vi "AuMT8852B AFH Scale.vi"(5 "Scale Factor (10)":enum16{"10", "20", "50", "100"}(ring), 7 "Set/Get (Set)":enum16{"Set", "Get"}(ring)=enum."Get", 8 "error in (no error)":errorcluster, 11 "VISA session":refnum<visa-resource-name>) -> (0 "error out":errorcluster, 2 "error code":i32, 3 "VISA session out":refnum<visa-resource-name>, 4 "Scale Factor out":enum16{"10", "20", "50", "100"}(ring))   [LabVIEW 2017]
doc: "Anritsu MT8852B Bluetooth Tester\n\nControls the scale value used for the \"chart recorder\" display when measuring channel utilisation or FER.\n\nINPUTS\nSet/Get - whether the value is being sent to or retrieved from the instrument.\nScale Factor - chart recorder display scale factor (10, 20, 50 and 100) setting.\n\nOUTPUTS\nScale Factor out - current chart recorder display scale setting."
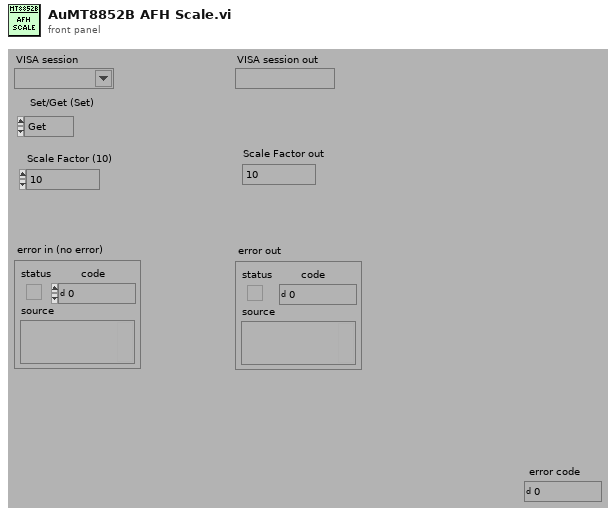
[diagram p1: front panel]
types:
  T1 = enum16{"Simulate", "Range check", "Cache", "Query instrument status"}
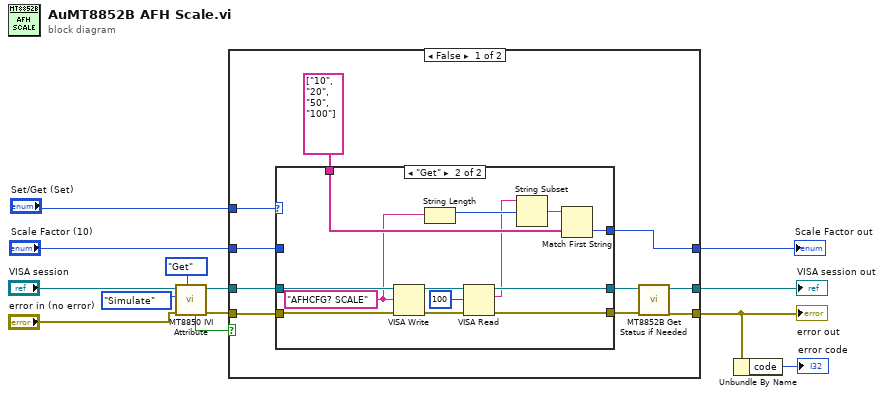
[diagram p0: block diagram]
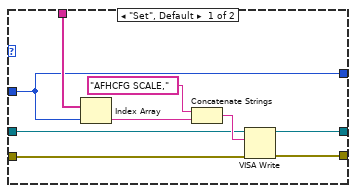
[diagram p2: hidden frame]
diagram:
  n1 = call <instrlib>:"MT8850 IVI Attribute.vi"("Set/Get (Set)"=enum16{"Set", "Get"}."Get", "error in (no error)"="error in (no error)", "Flag (Simulate)"=T1."Simulate", "VISA session"="VISA session") -> ("error out"=w12:errorcluster, "VISA session out"=w13:refnum<visa-resource-name>, "Value out"=w9:bool)  [unwired: 5 in]
  n2 = case shown="False" w9 {
    tunnel: [w18 w48] -> w7
    tunnel: [w19 w47] -> w6
    tunnel: w13 -> [w20 w48]
    tunnel: w12 -> [w21 w47]
    tunnel: [w22 w46] -> w3
    tunnel: "Scale Factor (10)" -> [w15 w46]
    tunnel: "Set/Get (Set)" -> [w14 _]
    frame False {
      n3 = case shown="\"Get\"" w14 {
        tunnel: string[] ["10", "20", "50", "100"] -> [w32 w42]
        tunnel: w15 -> [w28 _]
        tunnel: [w28 w41] -> w22
        tunnel: [w24 w38] -> w16
        tunnel: [w25 w37] -> w17
        tunnel: w21 -> [w27 w40]
        tunnel: w20 -> [w26 w39]
        frame "Set", Default {
          n4 = Index Array(array=w32, index=w28) -> (element=w31:string)
          n5 = Concatenate Strings("AFHCFG SCALE," ("write buffer (\"\")"), w31) -> (w29:string)
          n6 = VISA Write(VISA resource name=w26, write buffer=w29, error in (no error)=w27) -> (VISA resource name out=w25:refnum<visa-resource-name>, error out=w24:errorcluster)  [unwired: 1 out]
        }
        frame "Get" {
          w36 = "AFHCFG? SCALE" ("write buffer (\"\")")
          n7 = VISA Write(VISA resource name=w39, write buffer=w36, error in (no error)=w40) -> (VISA resource name out=w44:refnum<visa-resource-name>, error out=w45:errorcluster)  [unwired: 1 out]
          n8 = String Length(string=w36) -> (length=w34:i32)
          n9 = VISA Read(VISA resource name=w44, byte count=u32 100 ("byte count (0)"), error in (no error)=w45) -> (VISA resource name out=w37:refnum<visa-resource-name>, read buffer=w33:string, error out=w38:errorcluster)  [unwired: 1 out]
          n10 = String Subset(string=w33, offset (0)=w34) -> (substring=w35:string)  [unwired: 1 in]
          n11 = Match First String(2:w42, 3:w35) -> (0:w41:i32)  [unwired: 1 out]
        }
      }
      n12 = call <instrlib>:"MT8852B Get Status if Needed.vi"("error in (no error)"=w16, "VISA session"=w17) -> ("error out"=w19:errorcluster, "VISA session out"=w18:refnum<visa-resource-name>)  [unwired: 8 in]
    }
    frame True {
    }
  }
  "error out" <- w6
  "VISA session out" <- w7
  "Scale Factor out" <- w3
  n13 = Unbundle By Name(w6) -> ("code"=→"error code":i32)
